vi "Do Request.vi"(7 "Processing In":refnum<class "Processing.lvclass">, 11 "TestAuthController in":refnum<class "TestAuthController.lvclass">) -> (0 "error out":errorcluster, 5 "Processing":refnum<class "Processing.lvclass">)   [LabVIEW 2020, in "TestAuthController.lvclass"]
uses:
  TestAuthController.lvclass
  TestAuthController.lvclass/TestAuthController.ctl
  <vilib>/IlluminatedG/IG HTTP Server/HTTP Server/HTTP Server.lvlib
  <vilib>/IlluminatedG/IG HTTP Utils/HTTP Utils/Response/Response.lvclass
  TestUser/TestUser.lvclass
  <vilib>/IlluminatedG/IG HTTP Server/HTTP Server/Security/Security.lvclass
  <vilib>/IlluminatedG/IG HTTP Server/HTTP Server/Processing/Processing.lvclass
  C:/Program Files (x86)/National Instruments/LabVIEW 2020/vi.lib/IlluminatedG/IG HTTP Server/HTTP Server/Security/Security.lvclass
  C:/Program Files (x86)/National Instruments/LabVIEW 2020/vi.lib/IlluminatedG/IG HTTP Server/HTTP Server/Service/Service.lvclass
  C:/Program Files (x86)/National Instruments/LabVIEW 2020/vi.lib/IlluminatedG/IG HTTP Server/HTTP Server/User/User.lvclass
  C:/dev/lv 2020/lv-http-server-examples/Examples/TestUser/TestUser.lvclass
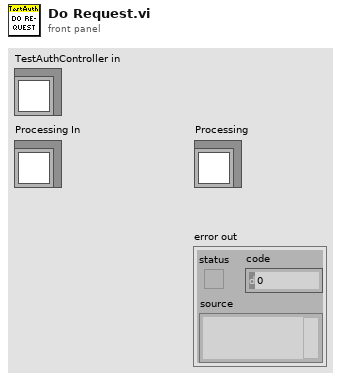
[diagram p1: front panel]
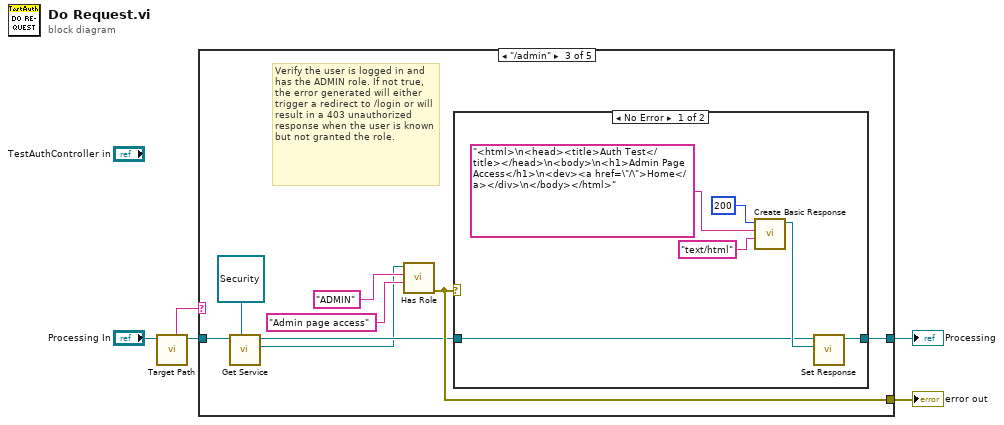
[diagram p0: block diagram]
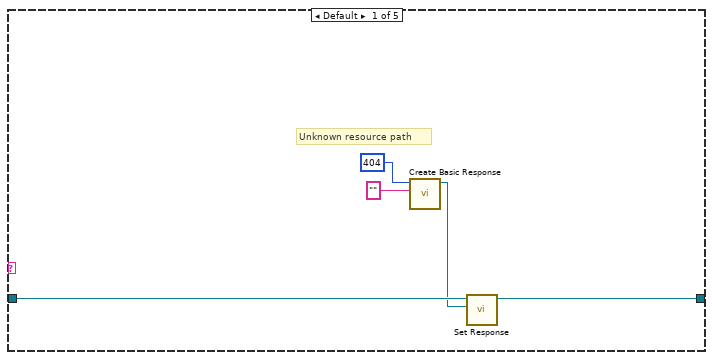
[diagram p2: hidden frame]
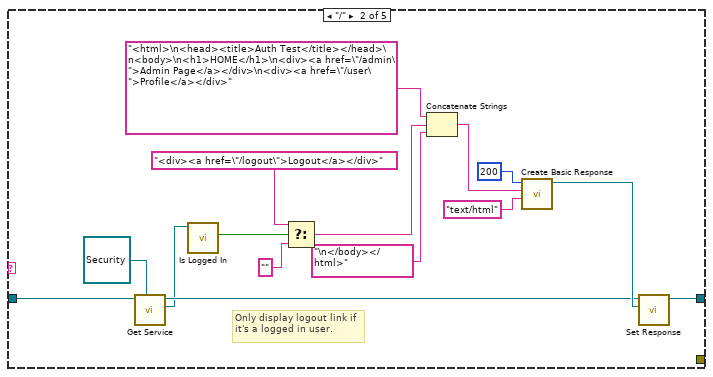
[diagram p3: hidden frame]
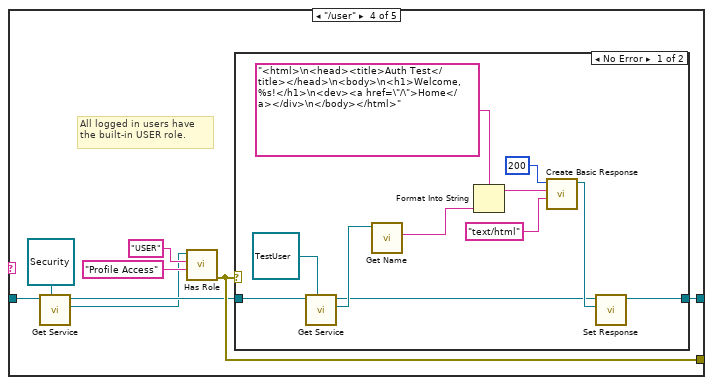
[diagram p5: hidden frame]
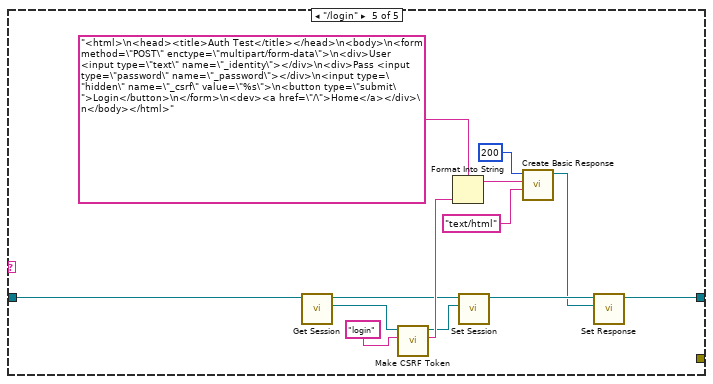
[diagram p7: hidden frame]
diagram:
  n1 = call <vilib>:"Target Path.vi"("Processing in"="Processing In") -> ("Processing out"=w3:refnum<class "Processing.lvclass">, "Target Path"=w4:string)  [unwired: 9 in]
  n2 = case shown="\"/admin\"" w4 {
    tunnel: [_ _ w31 w46 _] -> w5
    tunnel: [w6 w16 w30 w44 w62] -> w2
    tunnel: w3 -> [w8 w15 w29 w45 w63]
    frame Default {
      # "Unknown resource path"
      n3 = call <vilib>:"Create Basic Response.vi"("Payload"="", "Status Code"=u16 404) -> ("Response out"=w7:refnum<class "Response.lvclass">)  [unwired: 8 in, 1 out]
      n4 = call <vilib>:"Set Response.vi"("Response"=w7, "Processing in"=w8) -> ("Processing out"=w6:refnum<class "Processing.lvclass">)  [unwired: 9 in]
    }
    frame "/" {
      # "Only display logout link if it's a logged in user."
      n5 = call <vilib>:"Get Service.vi"("Service Type"=refnum<class "Security.lvclass"> refnum ("Security in"), "Processing in"=w15) -> ("Service"=w11:refnum<class "Security.lvclass">, "Processing out"=w13:refnum<class "Processing.lvclass">)  [unwired: 7 in, 1 out]
      n6 = call <vilib>:"Is Logged In.vi"("Security in"=w11) -> ("Logged In"=w17:bool)  [unwired: 8 in, 2 out]
      n7 = Select(t="<div><a href=\"/logout\">Logout</a></div>", s=w17, f="") -> (s? t:f=w18:string)
      n8 = Concatenate Strings("<html>\n<head><title>Auth Test</title></head>\n<body>\n<h1>HOME</h1>\n<div><a href=\"/admin\">Admin Page</a></div>\n<div><a href=\"/user\">Profile</a></div>", w18, "\n</body></html>") -> (w21:string)
      n9 = call <vilib>:"Create Basic Response.vi"("Content-Type (text/plain)"="text/html", "Payload"=w21, "Status Code"=u16 200) -> ("Response out"=w14:refnum<class "Response.lvclass">)  [unwired: 7 in, 1 out]
      n10 = call <vilib>:"Set Response.vi"("Response"=w14, "Processing in"=w13) -> ("Processing out"=w16:refnum<class "Processing.lvclass">)  [unwired: 9 in]
    }
    frame "/admin" {
      # "Verify the user is logged in and has the ADMIN role. If not true, the error generated will either trigger a redirect to /login or will result in a 403 unauthorized response when the user is known but not granted the role."
      n11 = call <vilib>:"Get Service.vi"("Service Type"=refnum<class "Security.lvclass"> refnum ("HTTP Server.lvlib:Security.lvclass"), "Processing in"=w29) -> ("Service"=w26:refnum<class "Security.lvclass">, "Processing out"=w28:refnum<class "Processing.lvclass">)  [unwired: 7 in, 1 out]
      n12 = call <vilib>:"Has Role.vi"("Description (None)"="Admin page access", "Role"="ADMIN", "Security in"=w26) -> ("error out"=w31:errorcluster)  [unwired: 6 in, 2 out]
      n13 = case shown="No Error" w31 {
        tunnel: [w36 w40] -> w30
        tunnel: w28 -> [w34 w40]
        frame No Error {
          n14 = call <vilib>:"Create Basic Response.vi"("Content-Type (text/plain)"="text/html", "Payload"="<html>\n<head><title>Auth Test</title></head>\n<body>\n<h1>Admin Page Access</h1>\n<dev><a href=\"/\">Home</a></div>\n</body></html>", "Status Code"=u16 200) -> ("Response out"=w35:refnum<class "Response.lvclass">)  [unwired: 7 in, 1 out]
          n15 = call <vilib>:"Set Response.vi"("Response"=w35, "Processing in"=w34) -> ("Processing out"=w36:refnum<class "Processing.lvclass">)  [unwired: 9 in]
        }
        frame Error {
        }
      }
    }
    frame "/user" {
      # "All logged in users have the built-in USER role."
      n16 = call <vilib>:"Get Service.vi"("Service Type"=refnum<class "Security.lvclass"> refnum ("HTTP Server.lvlib:Security.lvclass"), "Processing in"=w45) -> ("Service"=w42:refnum<class "Security.lvclass">, "Processing out"=w43:refnum<class "Processing.lvclass">)  [unwired: 7 in, 1 out]
      n17 = call <vilib>:"Has Role.vi"("Description (None)"="Profile Access", "Role"="USER", "Security in"=w42) -> ("error out"=w46:errorcluster)  [unwired: 6 in, 2 out]
      n18 = case shown="No Error" w46 {
        tunnel: w43 -> [w52 w60]
        tunnel: [w53 w60] -> w44
        frame No Error {
          n19 = call <vilib>:"Get Service.vi"("Service Type"=refnum<class "TestUser.lvclass"> refnum ("TestUser.lvclass"), "Processing in"=w52) -> ("Service"=w50:refnum<class "TestUser.lvclass">, "Processing out"=w49:refnum<class "Processing.lvclass">)  [unwired: 7 in, 1 out]
          n20 = call "Get Name.vi"("TestUser in"=w50) -> ("Name"=w59:string)  [unwired: 8 in, 2 out]
          n21 = Format Into String(format string="<html>\n<head><title>Auth Test</title></head>\n<body>\n<h1>Welcome, %s!</h1>\n<dev><a href=\"/\">Home</a></div>\n</body></html>", w59) -> (resulting string=w58:string)  [unwired: 2 in, 1 out]
          n22 = call <vilib>:"Create Basic Response.vi"("Content-Type (text/plain)"="text/html", "Payload"=w58, "Status Code"=u16 200) -> ("Response out"=w54:refnum<class "Response.lvclass">)  [unwired: 7 in, 1 out]
          n23 = call <vilib>:"Set Response.vi"("Response"=w54, "Processing in"=w49) -> ("Processing out"=w53:refnum<class "Processing.lvclass">)  [unwired: 9 in]
        }
        frame Error {
        }
      }
    }
    frame "/login" {
      n24 = call <vilib>:"Get Session.vi"("Processing in"=w63) -> ("Session"=w67:refnum<class "Session.lvclass">, "Processing out"=w66:refnum<class "Processing.lvclass">)  [unwired: 9 in]
      n25 = call <vilib>:"Make CSRF Token.vi"("Token ID"="login", "Session In"=w67) -> ("Token"=w71:string, "Session"=w65:refnum<class "Session.lvclass">)  [unwired: 7 in, 1 out]
      n26 = Format Into String(format string="<html>\n<head><title>Auth Test</title></head>\n<body>\n<form method=\"POST\" enctype=\"multipart/form-data\">\n<div>User <input type=\"text\" name=\"_identity\"></div>\n<div>Pass <input type=\"password\" name=\"_password\"></div>\n<input type=\"hidden\" name=\"_csrf\" value=\"%s\">\n<button type=\"submit\">Login</button>\n</form>\n<dev><a href=\"/\">Home</a></div>\n</body></html>", w71) -> (resulting string=w70:string)  [unwired: 2 in, 1 out]
      n27 = call <vilib>:"Set Session.vi"("Session"=w65, "Processing in"=w66) -> ("Processing out"=w64:refnum<class "Processing.lvclass">)  [unwired: 9 in]
      n28 = call <vilib>:"Create Basic Response.vi"("Content-Type (text/plain)"="text/html", "Payload"=w70, "Status Code"=u16 200) -> ("Response out"=w61:refnum<class "Response.lvclass">)  [unwired: 7 in, 1 out]
      n29 = call <vilib>:"Set Response.vi"("Response"=w61, "Processing in"=w64) -> ("Processing out"=w62:refnum<class "Processing.lvclass">)  [unwired: 9 in]
    }
  }
  "error out" <- w5
  "Processing" <- w2
